vi "increment_laser_power.vi"(8 "error in":errorcluster, 9 "increment":dbl, 10 "manual laser power":dbl, 11 "heat output ref":refnum<k24>) -> (0 "error out":errorcluster, 3 "new manual laser power":dbl)   [LabVIEW 2015]
uses:
  C:/Program Files/National Instruments/LabVIEW 2015/vi.lib/ULx/ULx_LV.dll
  <vilib>/ULx/Write.llb/ULx Write (Analog 1D DBL 1Chan 1Samp).vi
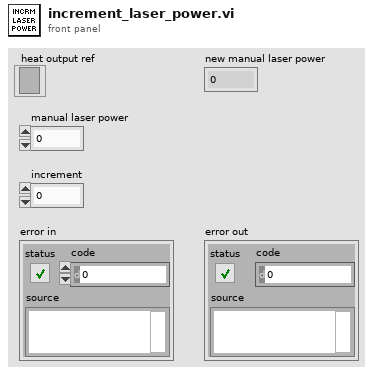
[diagram p1: front panel]
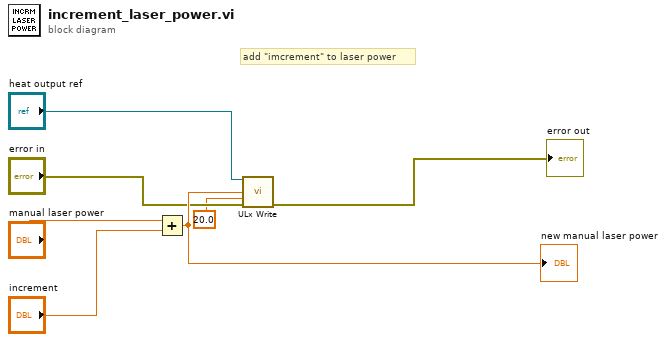
[diagram p0: block diagram]
diagram:
  # "add \"imcrement\" to laser power"
  n1 = Add(x="manual laser power", y="increment") -> (x+y=w7:dbl)
  "new manual laser power" <- w7
  n2 = call-poly <vilib>:"ULx Write.vi"("task in"="heat output ref", "data"=w7, "timeout"=20.0, "error in"="error in") -> ("error out"=→"error out":errorcluster)  [unwired: 9 in, 2 out]
